vi "Process Launcher.vi"(8 "error in (no error)":errorcluster, 11 "Process Queue ref":refnum<queue>) -> (0 "error out":errorcluster)   [LabVIEW 2020, in "Process.lvclass"]
uses:
  Process.lvclass
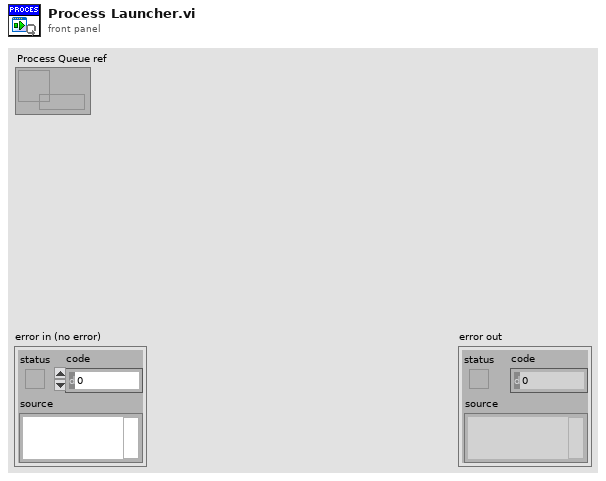
[diagram p1: front panel]
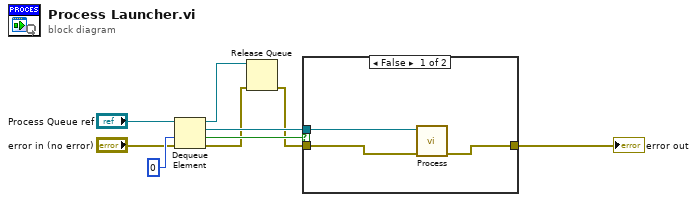
[diagram p0: block diagram]
diagram:
  n1 = Dequeue Element(queue="Process Queue ref", timeout in ms (-1)=0, error in (no error)="error in (no error)") -> (queue out=w4:refnum<queue>, element=w6:refnum<class "Process.lvclass">, timed out?=w7:bool, error out=w3:errorcluster)
  n2 = Release Queue(queue=w4, error in (no error)=w3) -> (error out=w2:errorcluster)  [unwired: 1 in, 2 out]
  n3 = case shown="False" w7 {
    tunnel: w6 -> [w12 _]
    tunnel: w2 -> [w11 w13]
    tunnel: [w10 w13] -> w1
    frame False {
      n4 = call-dynamic "Process.vi"("error in (no error)"=w11, "Process In"=w12) -> ("error out"=w10:errorcluster)  [unwired: 8 in, 1 out]
    }
    frame True {
    }
  }
  "error out" <- w1
